vi "IKA_Eurostar60.vi"(5 "IKAenable":bool=TRUE, 6 "Timeout(s)":dbl=2.0, 7 "Command":T1, 8 "Error in":errorcluster, 9 "Set_parametro":dbl format="%.3f", 11 "VISA Paar mPDS2000":refnum<visa-resource-name>="ASRL6::INSTR") -> (0 "error out":errorcluster, 1 "Read_parametro":dbl format="%.3f", 2 "read string":string)   [LabVIEW 2017]
uses:
  IKA_Eurostar60.ctl
  <vilib>/Instr/_visa.llb/VISA Configure Serial Port (Instr).vi
panel:
  in  "EOS":string="\n"
  # "Input Data"
  # "Output Data"
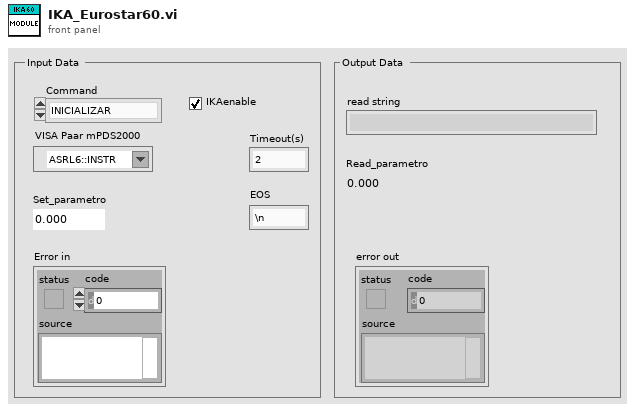
[diagram p1: front panel]
types:
  T1 = typedef "IKA_Eurostar60.ctl" = enum16{"INICIALIZAR", "READ NOMBRE APARATO", "READ VALOR PT100", "READ VELOCIDAD ACTUAL", "READ PAR DE GIRO ACTUAL", "READ VELOCIDAD NOMINAL", "READ LIMITE PAR DE GIRO", "READ LIMITE VELOCIDAD", "READ VELOCIDAD SEGURIDAD", "SET VELOCIDAD NOMINAL", "SET LIMITE PAR DE GIRO", "SET LIMITE VELOCIDAD", "SET VELOCIDAD SEGURIDAD", "ARRANCAR MOTOR", "DETENER MOTOR", "RESET", "SET SENTIDO DE GIRO", "READ SENTIDO DE GIRO", "FINALIZAR"}
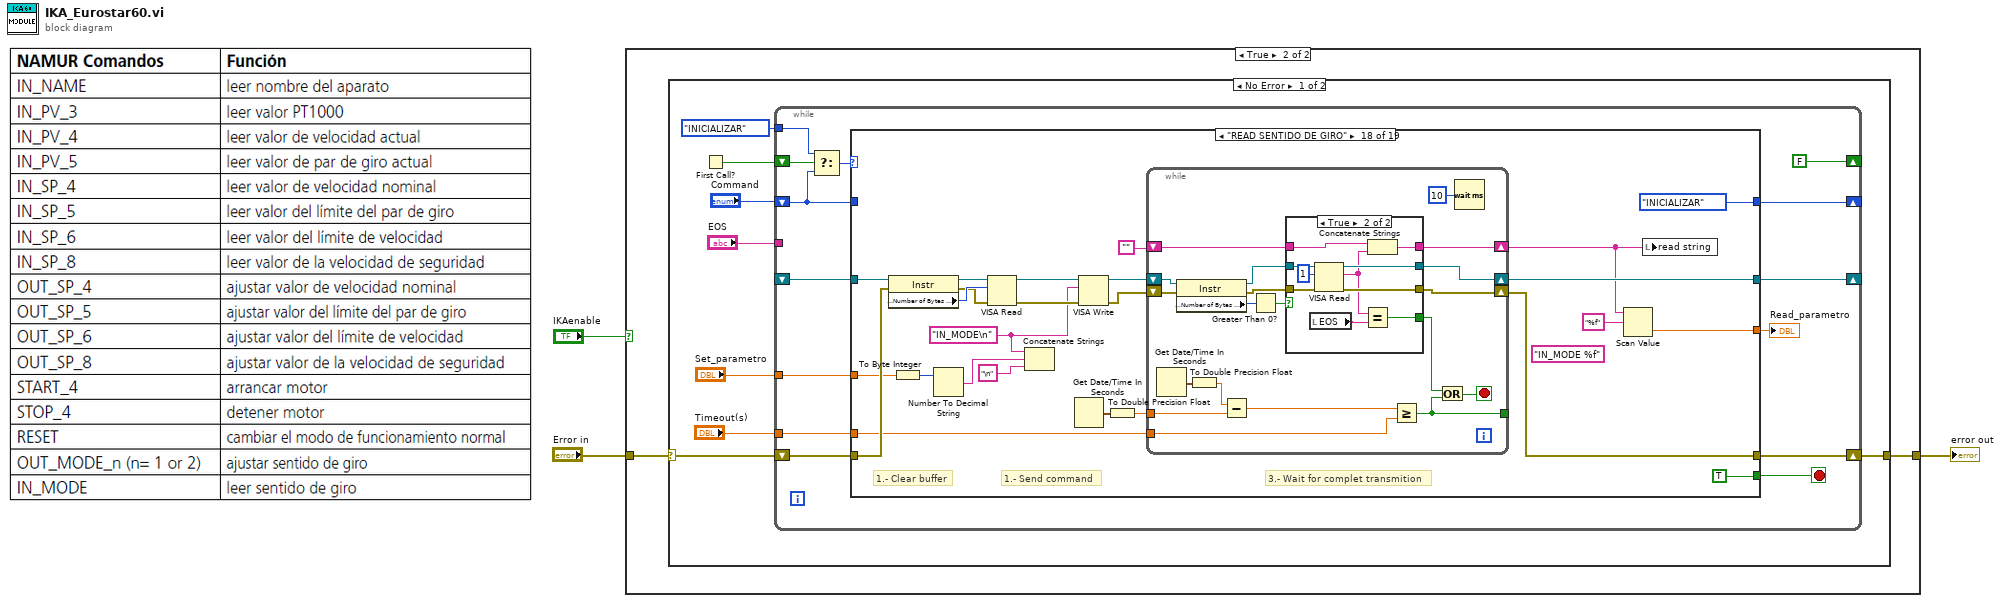
[diagram p0: block diagram]
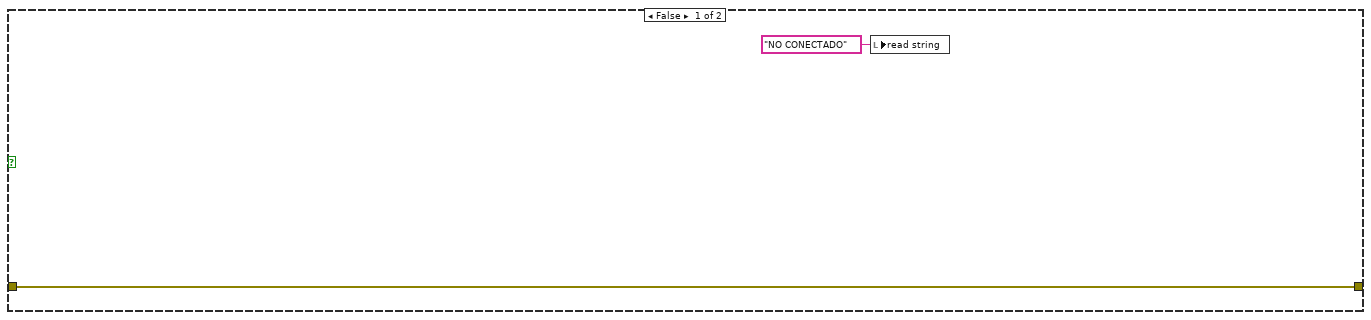
[diagram p2: hidden frame]
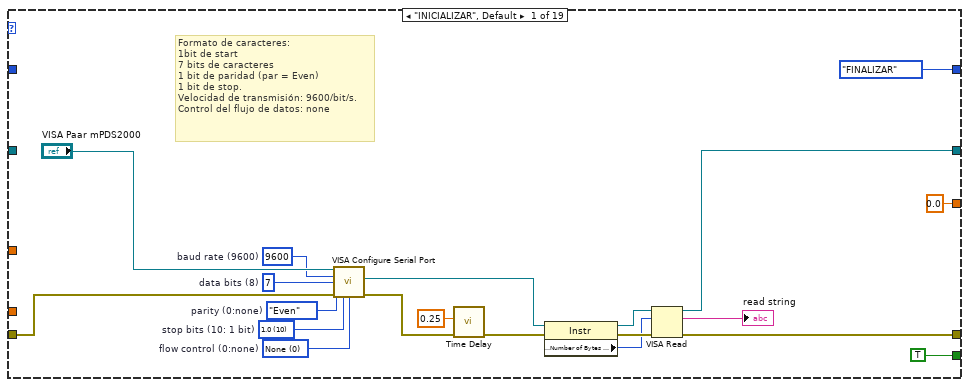
[diagram p3: hidden frame]
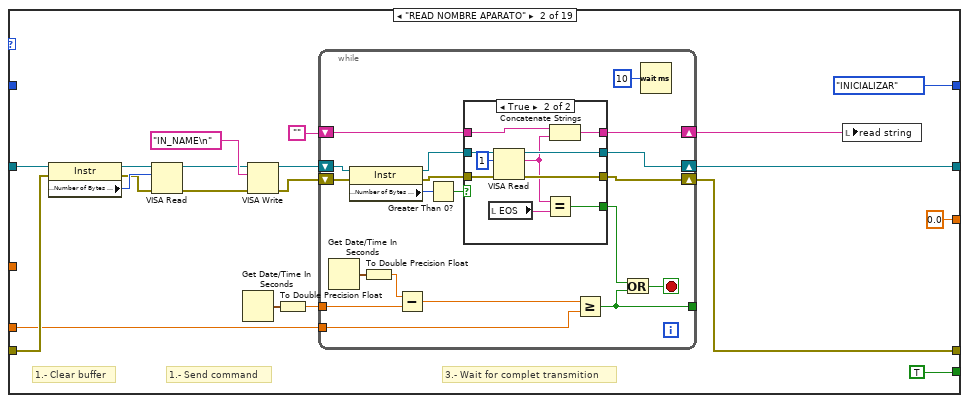
[diagram p4: hidden frame]
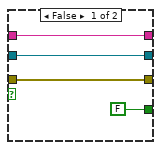
[diagram p5: hidden frame]
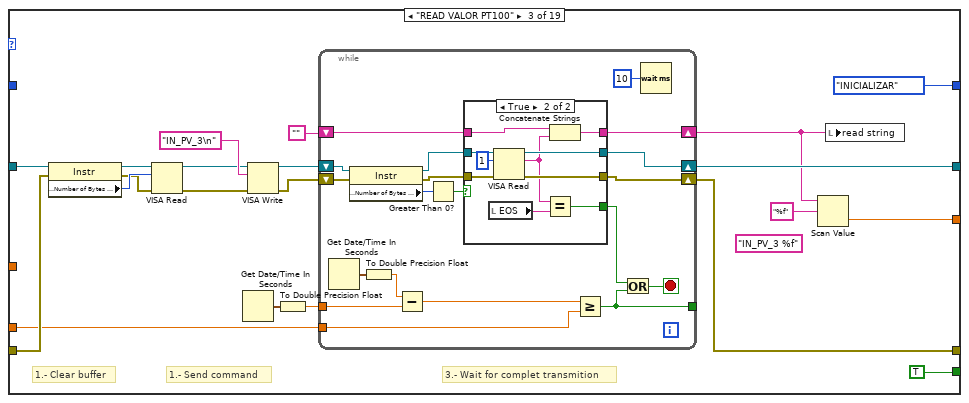
[diagram p6: hidden frame]
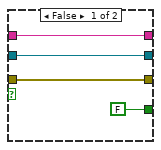
[diagram p7: hidden frame]
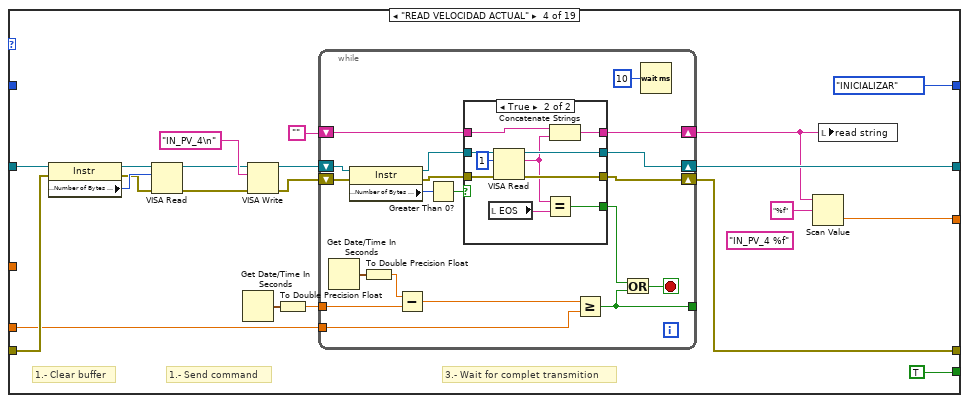
[diagram p8: hidden frame]
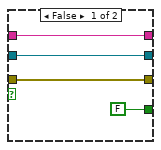
[diagram p9: hidden frame]
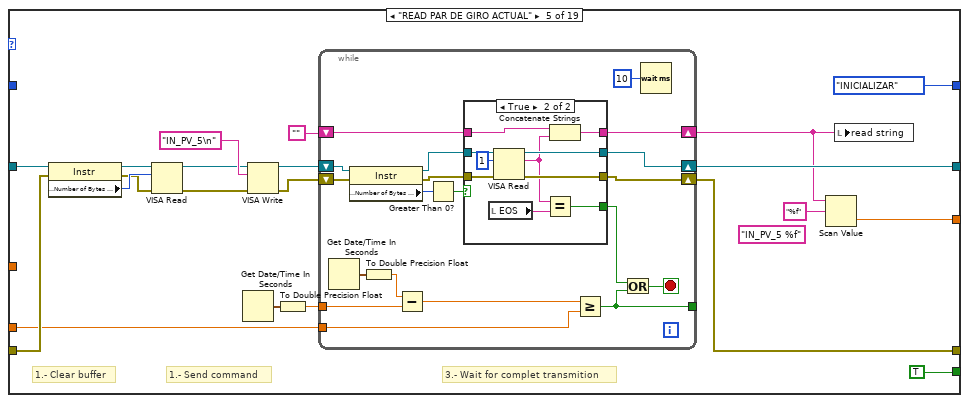
[diagram p10: hidden frame]
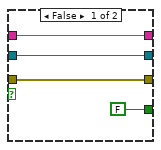
[diagram p11: hidden frame]
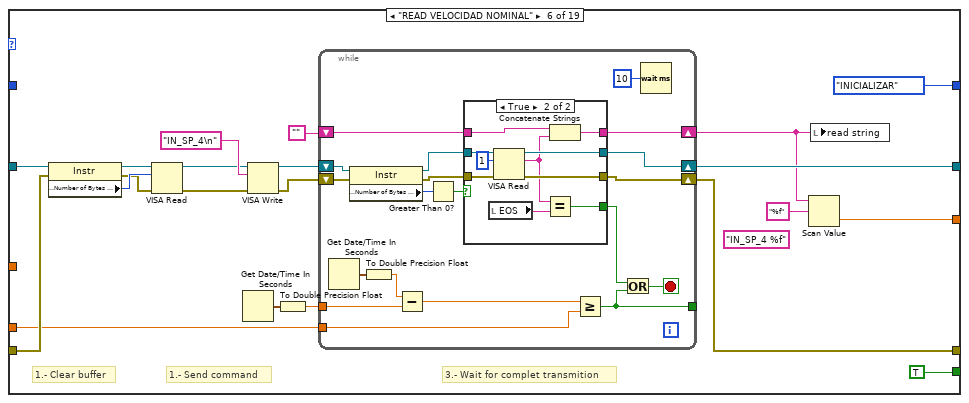
[diagram p12: hidden frame]
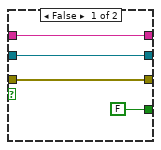
[diagram p13: hidden frame]
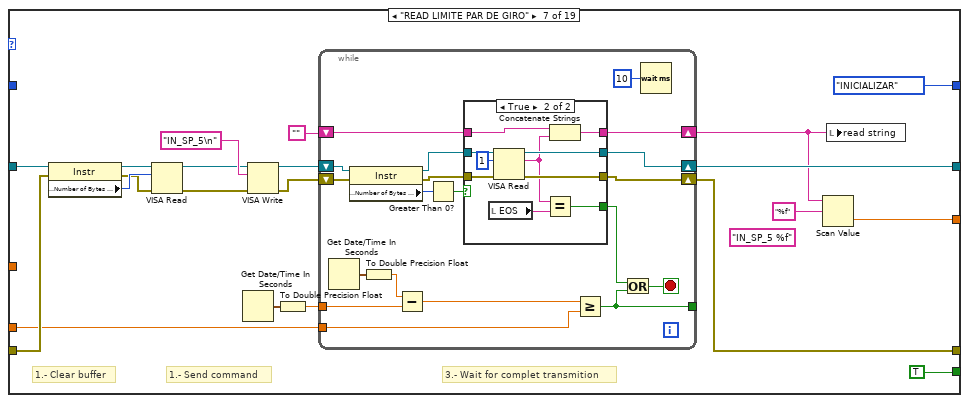
[diagram p14: hidden frame]
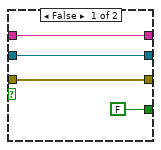
[diagram p15: hidden frame]
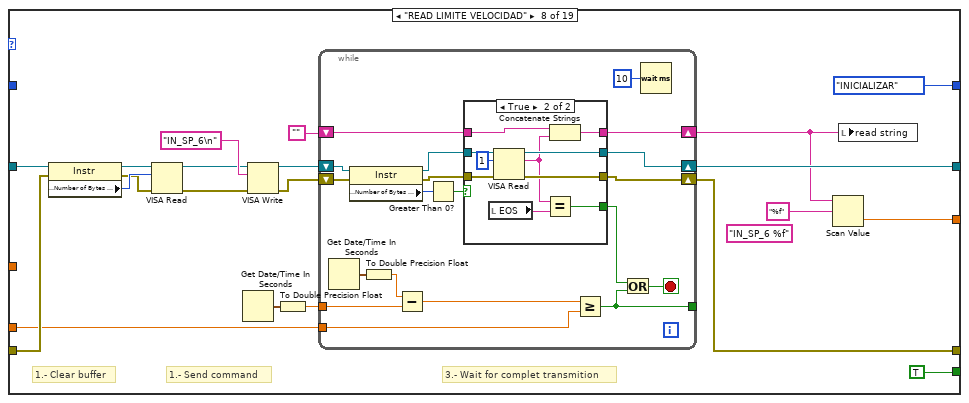
[diagram p16: hidden frame]
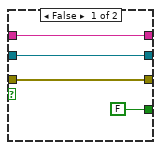
[diagram p17: hidden frame]
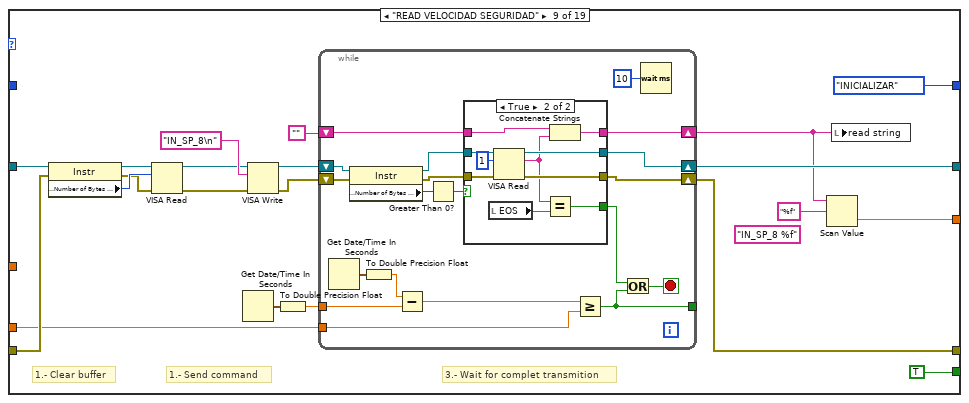
[diagram p18: hidden frame]
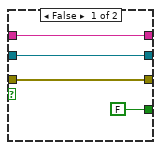
[diagram p19: hidden frame]
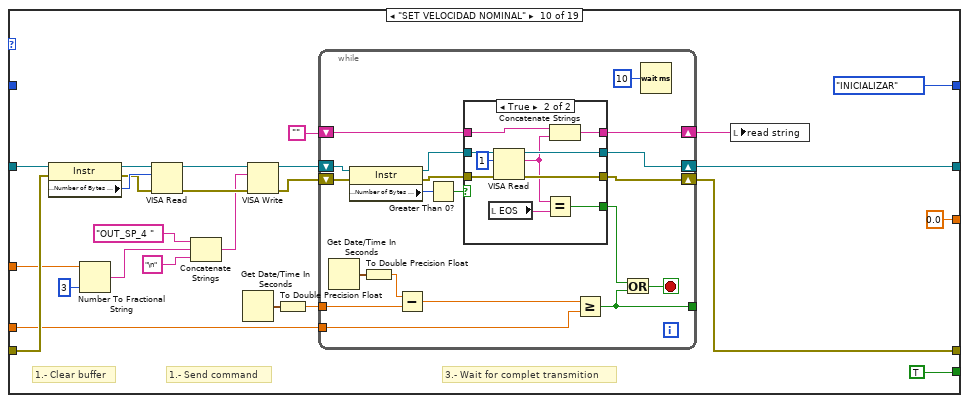
[diagram p20: hidden frame]
diagram:
  n1 = case shown="True" "IKAenable" {
    tunnel: "Error in" -> [w5 w7]
    tunnel: [w5 w6] -> w2
    frame False {
      n2 = local write "read string"("NO CONECTADO" ("read string")) -> ()
    }
    frame True {
      n3 = case shown="No Error" w7 {
        selector: w7 -> [w13 w1006]
        tunnel: [w12 w1006] -> w6
        frame No Error {
          n4 = First Call?() -> (First Call?: T/F=w15:bool)
          n5 = while {
            shift-right: [w21] -> _
            shift-left: "Command" -> [w22]
            shift-right: [w24] -> w12
            shift-left: w13 -> [w25]
            shift-right: [FALSE ("First Call?: T/F")] -> _
            shift-left: w15 -> [w29]
            tunnel: IKA_Eurostar60."INICIALIZAR" ("t") -> [w28]
            shift-right: [w19] -> _
            shift-left: _ -> [w20]
            tunnel: "Timeout(s)" -> [w18]
            tunnel: "Set_parametro" -> [w17]
            tunnel: "EOS" -> [_]
            stop <- w26 stop-if-true
            n6 = Select(t=w28, s=w29, f=w22) -> (s? t:f=w27:T1)
            n7 = case shown="\"READ SENTIDO DE GIRO\"" w27 {
              tunnel: [TRUE TRUE TRUE TRUE TRUE TRUE TRUE TRUE TRUE TRUE TRUE TRUE TRUE TRUE TRUE TRUE TRUE TRUE TRUE] -> w26
              tunnel: w25 -> [w46 w61 w115 w169 w223 w277 w331 w385 w439 w498 w556 w614 w672 w729 w786 w843 w901 w959 w1004]
              tunnel: [w48 w53 w107 w161 w215 w269 w323 w377 w431 w490 w548 w606 w664 w721 w778 w835 w893 w951 w1003] -> w24
              tunnel: w22 -> [_ _ _ _ _ _ _ _ _ _ _ _ _ _ _ _ _ _ _]
              tunnel: [IKA_Eurostar60."FINALIZAR" ("t") IKA_Eurostar60."INICIALIZAR" ("t") IKA_Eurostar60."INICIALIZAR" ("t") IKA_Eurostar60."INICIALIZAR" ("t") IKA_Eurostar60."INICIALIZAR" ("t") IKA_Eurostar60."INICIALIZAR" ("t") IKA_Eurostar60."INICIALIZAR" ("t") IKA_Eurostar60."INICIALIZAR" ("t") IKA_Eurostar60."INICIALIZAR" ("t") IKA_Eurostar60."INICIALIZAR" ("t") IKA_Eurostar60."INICIALIZAR" ("t") IKA_Eurostar60."INICIALIZAR" ("t") IKA_Eurostar60."INICIALIZAR" ("t") IKA_Eurostar60."INICIALIZAR" ("t") IKA_Eurostar60."INICIALIZAR" ("t") IKA_Eurostar60."INICIALIZAR" ("t") IKA_Eurostar60."INICIALIZAR" ("t") IKA_Eurostar60."INICIALIZAR" ("t") IKA_Eurostar60."FINALIZAR" ("t")] -> w21
              tunnel: w20 -> [_ w62 w116 w170 w224 w278 w332 w386 w440 w499 w557 w615 w673 w730 w787 w844 w902 w960 w1002]
              tunnel: [w47 w54 w108 w162 w216 w270 w324 w378 w432 w491 w549 w607 w665 w722 w779 w836 w894 w952 w1002] -> w19
              tunnel: w18 -> [_ w55 w109 w163 w217 w271 w325 w379 w433 w492 w550 w608 w666 w723 w780 w837 w895 w953 _]
              tunnel: w17 -> [_ _ _ _ _ _ _ _ _ w486 w544 w602 w660 w717 w774 w831 w888 w947 _]
              tunnel: [0.0 0.0 w103 w158 w211 w266 w321 w375 w427 0.0 0.0 0.0 0.0 0.0 0.0 0.0 0.0 w942 0.0] -> w16
              frame "INICIALIZAR", Default {
                w33 = u16 0 items=["None", "XON/XOFF", "RTS/CTS", "XON/XOFF & RTS/CTS", "DTR/DSR", "XON/XOFF & DTR/DSR"]  # flow control (0:none)
                w34 = u16 10 items=["1.0"=10, "1.5"=15, "2.0"=20]  # stop bits (10: 1 bit)
                w35 = enum16{"None", "Odd", "Even", "Mark", "Space"}."Even"  # parity (0:none)
                w36 = u16 7  # data bits (8)
                w37 = u32 9600  # baud rate (9600)
                # "Formato de caracteres: \n1bit de start\n7 bits de caracteres\n1 bit de paridad (par = Even)\n1 bit de stop.\nVelocidad de transmisión: 9600/bit/s.\nControl del flujo de datos: none"
                n8 = call-poly "VISA Configure Serial Port"("VISA resource name"="VISA Paar mPDS2000", "baud rate (9600)"=w37, "data bits (8)"=w36, "parity (0:none)"=w35, "error in (no error)"=w46, "stop bits (10: 1 bit)"=w34, "flow control (0:none)"=w33) -> ("VISA resource name out"=w41:refnum<visa-resource-name>, "error out"=w39:errorcluster)  [unwired: 7 in]
                n9 = call "Time Delay"("error in (no error)"=w39, "Delay Time (s)"=0.25) -> ("error out"=w38:errorcluster)  [unwired: 9 in]
                n10 = property class="Instr"(reference=w41, error in=w38) -> (reference out=w44:refnum<visa-resource-name>, error out=w43:errorcluster, "Serial Settings:Number of Bytes at Serial Port"=w42:u32)
                n11 = VISA Read(VISA resource name=w44, byte count=w42, error in (no error)=w43) -> (VISA resource name out=w47:refnum<visa-resource-name>, read buffer=→"read string":string, error out=w48:errorcluster)  [unwired: 1 out]
              }
              frame "READ NOMBRE APARATO" {
                # "1.- Send command"
                # "3.- Wait for complet transmition"
                # "1.- Clear buffer"
                n12 = property class="Instr"(reference=w62, error in=w61) -> (reference out=w65:refnum<visa-resource-name>, error out=w66:errorcluster, "Serial Settings:Number of Bytes at Serial Port"=w67:u32)
                n13 = VISA Read(VISA resource name=w65, byte count=w67, error in (no error)=w66) -> (VISA resource name out=w64:refnum<visa-resource-name>, error out=w63:errorcluster)  [unwired: 2 out]
                n14 = Get Date/Time In Seconds() -> (seconds since 1Jan1904=w59:timestamp)
                n15 = VISA Write(VISA resource name=w64, write buffer="IN_NAME\n" ("Mide"), error in (no error)=w63) -> (VISA resource name out=w57:refnum<visa-resource-name>, error out=w56:errorcluster)  [unwired: 1 out]
                n16 = To Double Precision Float(number=w59) -> (double precision float=w58:dbl)
                n17 = while {
                  tunnel: w58 -> [w85]
                  shift-right: [w73] -> w54
                  shift-left: w57 -> [w84]
                  shift-right: [w72] -> w53
                  shift-left: w56 -> [w83]
                  tunnel: w55 -> [w81]
                  tunnel: [w80] -> _
                  shift-right: [w76] -> w51
                  shift-left: "" -> [w71]
                  stop <- w88 stop-if-true
                  n18 = Get Date/Time In Seconds() -> (seconds since 1Jan1904=w87:timestamp)
                  n19 = property class="Instr"(reference=w84, error in=w83) -> (reference out=w74:refnum<visa-resource-name>, error out=w75:errorcluster, "Serial Settings:Number of Bytes at Serial Port"=w78:u32)
                  n20 = To Double Precision Float(number=w87) -> (double precision float=w86:dbl)
                  n21 = Subtract(x=w86, y=w85) -> (x-y=w82:dbl)
                  n22 = Greater Than 0?(x=w78) -> (x > 0?=w77:bool)
                  n23 = case shown="True" w77 {
                    tunnel: w71 -> [w92 w97]
                    tunnel: [w92 w96] -> w76
                    tunnel: w75 -> [w90 w102]
                    tunnel: w74 -> [w89 w101]
                    tunnel: [w89 w100] -> w73
                    tunnel: [w90 w99] -> w72
                    tunnel: [FALSE w94] -> w70
                    frame False {
                    }
                    frame True {
                      n24 = local read "EOS"() -> (w93:string)
                      n25 = VISA Read(VISA resource name=w101, byte count=u32 1, error in (no error)=w102) -> (VISA resource name out=w100:refnum<visa-resource-name>, read buffer=w95:string, error out=w99:errorcluster)  [unwired: 1 out]
                      n26 = Equal?(x=w95, y=w93) -> (x = y?=w94:bool)
                      n27 = Concatenate Strings(w97, w95) -> (w96:string)
                    }
                  }
                  n28 = Greater Or Equal?(x=w82, y=w81) -> (x >= y?=w80:bool)
                  n29 = Or(x=w70, y=w80) -> (x .or. y?=w88:bool)
                  n30 = Wait (ms)(milliseconds to wait=u32 10) -> ()  [unwired: 1 out]
                }
                n31 = local write "read string"(w51) -> ()
              }
              frame "READ VALOR PT100" {
                (unwired) "IN_PV_3 %f" ("format string")
                # "1.- Send command"
                # "3.- Wait for complet transmition"
                # "1.- Clear buffer"
                n32 = property class="Instr"(reference=w116, error in=w115) -> (reference out=w119:refnum<visa-resource-name>, error out=w120:errorcluster, "Serial Settings:Number of Bytes at Serial Port"=w121:u32)
                n33 = VISA Read(VISA resource name=w119, byte count=w121, error in (no error)=w120) -> (VISA resource name out=w118:refnum<visa-resource-name>, error out=w117:errorcluster)  [unwired: 2 out]
                n34 = Get Date/Time In Seconds() -> (seconds since 1Jan1904=w113:timestamp)
                n35 = VISA Write(VISA resource name=w118, write buffer="IN_PV_3\n" ("Mide"), error in (no error)=w117) -> (VISA resource name out=w111:refnum<visa-resource-name>, error out=w110:errorcluster)  [unwired: 1 out]
                n36 = To Double Precision Float(number=w113) -> (double precision float=w112:dbl)
                n37 = while {
                  tunnel: w112 -> [w139]
                  shift-right: [w127] -> w108
                  shift-left: w111 -> [w138]
                  shift-right: [w126] -> w107
                  shift-left: w110 -> [w137]
                  tunnel: w109 -> [w135]
                  tunnel: [w134] -> _
                  shift-right: [w130] -> w104
                  shift-left: "" -> [w125]
                  stop <- w142 stop-if-true
                  n38 = Get Date/Time In Seconds() -> (seconds since 1Jan1904=w141:timestamp)
                  n39 = property class="Instr"(reference=w138, error in=w137) -> (reference out=w128:refnum<visa-resource-name>, error out=w129:errorcluster, "Serial Settings:Number of Bytes at Serial Port"=w132:u32)
                  n40 = To Double Precision Float(number=w141) -> (double precision float=w140:dbl)
                  n41 = Subtract(x=w140, y=w139) -> (x-y=w136:dbl)
                  n42 = Greater Than 0?(x=w132) -> (x > 0?=w131:bool)
                  n43 = case shown="True" w131 {
                    tunnel: w125 -> [w146 w151]
                    tunnel: [w146 w150] -> w130
                    tunnel: w129 -> [w144 w156]
                    tunnel: w128 -> [w143 w155]
                    tunnel: [w143 w154] -> w127
                    tunnel: [w144 w153] -> w126
                    tunnel: [FALSE w148] -> w124
                    frame False {
                    }
                    frame True {
                      n44 = local read "EOS"() -> (w147:string)
                      n45 = VISA Read(VISA resource name=w155, byte count=u32 1, error in (no error)=w156) -> (VISA resource name out=w154:refnum<visa-resource-name>, read buffer=w149:string, error out=w153:errorcluster)  [unwired: 1 out]
                      n46 = Equal?(x=w149, y=w147) -> (x = y?=w148:bool)
                      n47 = Concatenate Strings(w151, w149) -> (w150:string)
                    }
                  }
                  n48 = Greater Or Equal?(x=w136, y=w135) -> (x >= y?=w134:bool)
                  n49 = Or(x=w124, y=w134) -> (x .or. y?=w142:bool)
                  n50 = Wait (ms)(milliseconds to wait=u32 10) -> ()  [unwired: 1 out]
                }
                n51 = Scan Value(string=w104, format string="%f") -> (value=w103:dbl)  [unwired: 1 in, 1 out]
                n52 = local write "read string"(w104) -> ()
              }
              frame "READ VELOCIDAD ACTUAL" {
                (unwired) "IN_PV_4 %f" ("format string")
                # "1.- Send command"
                # "3.- Wait for complet transmition"
                # "1.- Clear buffer"
                n53 = property class="Instr"(reference=w170, error in=w169) -> (reference out=w173:refnum<visa-resource-name>, error out=w174:errorcluster, "Serial Settings:Number of Bytes at Serial Port"=w175:u32)
                n54 = VISA Read(VISA resource name=w173, byte count=w175, error in (no error)=w174) -> (VISA resource name out=w172:refnum<visa-resource-name>, error out=w171:errorcluster)  [unwired: 2 out]
                n55 = Get Date/Time In Seconds() -> (seconds since 1Jan1904=w167:timestamp)
                n56 = VISA Write(VISA resource name=w172, write buffer="IN_PV_4\n" ("Mide"), error in (no error)=w171) -> (VISA resource name out=w165:refnum<visa-resource-name>, error out=w164:errorcluster)  [unwired: 1 out]
                n57 = To Double Precision Float(number=w167) -> (double precision float=w166:dbl)
                n58 = while {
                  tunnel: w166 -> [w193]
                  shift-right: [w181] -> w162
                  shift-left: w165 -> [w192]
                  shift-right: [w180] -> w161
                  shift-left: w164 -> [w191]
                  tunnel: w163 -> [w189]
                  tunnel: [w188] -> _
                  shift-right: [w184] -> w157
                  shift-left: "" -> [w179]
                  stop <- w196 stop-if-true
                  n59 = Get Date/Time In Seconds() -> (seconds since 1Jan1904=w195:timestamp)
                  n60 = property class="Instr"(reference=w192, error in=w191) -> (reference out=w182:refnum<visa-resource-name>, error out=w183:errorcluster, "Serial Settings:Number of Bytes at Serial Port"=w186:u32)
                  n61 = To Double Precision Float(number=w195) -> (double precision float=w194:dbl)
                  n62 = Subtract(x=w194, y=w193) -> (x-y=w190:dbl)
                  n63 = Greater Than 0?(x=w186) -> (x > 0?=w185:bool)
                  n64 = case shown="True" w185 {
                    tunnel: w179 -> [w200 w205]
                    tunnel: [w200 w204] -> w184
                    tunnel: w183 -> [w198 w210]
                    tunnel: w182 -> [w197 w209]
                    tunnel: [w197 w208] -> w181
                    tunnel: [w198 w207] -> w180
                    tunnel: [FALSE w202] -> w178
                    frame False {
                    }
                    frame True {
                      n65 = local read "EOS"() -> (w201:string)
                      n66 = VISA Read(VISA resource name=w209, byte count=u32 1, error in (no error)=w210) -> (VISA resource name out=w208:refnum<visa-resource-name>, read buffer=w203:string, error out=w207:errorcluster)  [unwired: 1 out]
                      n67 = Equal?(x=w203, y=w201) -> (x = y?=w202:bool)
                      n68 = Concatenate Strings(w205, w203) -> (w204:string)
                    }
                  }
                  n69 = Greater Or Equal?(x=w190, y=w189) -> (x >= y?=w188:bool)
                  n70 = Or(x=w178, y=w188) -> (x .or. y?=w196:bool)
                  n71 = Wait (ms)(milliseconds to wait=u32 10) -> ()  [unwired: 1 out]
                }
                n72 = Scan Value(string=w157, format string="%f") -> (value=w158:dbl)  [unwired: 1 in, 1 out]
                n73 = local write "read string"(w157) -> ()
              }
              frame "READ PAR DE GIRO ACTUAL" {
                (unwired) "IN_PV_5 %f" ("format string")
                # "1.- Send command"
                # "3.- Wait for complet transmition"
                # "1.- Clear buffer"
                n74 = property class="Instr"(reference=w224, error in=w223) -> (reference out=w227:refnum<visa-resource-name>, error out=w228:errorcluster, "Serial Settings:Number of Bytes at Serial Port"=w229:u32)
                n75 = VISA Read(VISA resource name=w227, byte count=w229, error in (no error)=w228) -> (VISA resource name out=w226:refnum<visa-resource-name>, error out=w225:errorcluster)  [unwired: 2 out]
                n76 = Get Date/Time In Seconds() -> (seconds since 1Jan1904=w221:timestamp)
                n77 = VISA Write(VISA resource name=w226, write buffer="IN_PV_5\n" ("Mide"), error in (no error)=w225) -> (VISA resource name out=w219:refnum<visa-resource-name>, error out=w218:errorcluster)  [unwired: 1 out]
                n78 = To Double Precision Float(number=w221) -> (double precision float=w220:dbl)
                n79 = while {
                  tunnel: w220 -> [w247]
                  shift-right: [w235] -> w216
                  shift-left: w219 -> [w246]
                  shift-right: [w234] -> w215
                  shift-left: w218 -> [w245]
                  tunnel: w217 -> [w243]
                  tunnel: [w242] -> _
                  shift-right: [w238] -> w212
                  shift-left: "" -> [w233]
                  stop <- w250 stop-if-true
                  n80 = Get Date/Time In Seconds() -> (seconds since 1Jan1904=w249:timestamp)
                  n81 = property class="Instr"(reference=w246, error in=w245) -> (reference out=w236:refnum<visa-resource-name>, error out=w237:errorcluster, "Serial Settings:Number of Bytes at Serial Port"=w240:u32)
                  n82 = To Double Precision Float(number=w249) -> (double precision float=w248:dbl)
                  n83 = Subtract(x=w248, y=w247) -> (x-y=w244:dbl)
                  n84 = Greater Than 0?(x=w240) -> (x > 0?=w239:bool)
                  n85 = case shown="True" w239 {
                    tunnel: w233 -> [w254 w259]
                    tunnel: [w254 w258] -> w238
                    tunnel: w237 -> [w252 w264]
                    tunnel: w236 -> [w251 w263]
                    tunnel: [w251 w262] -> w235
                    tunnel: [w252 w261] -> w234
                    tunnel: [FALSE w256] -> w232
                    frame False {
                    }
                    frame True {
                      n86 = local read "EOS"() -> (w255:string)
                      n87 = VISA Read(VISA resource name=w263, byte count=u32 1, error in (no error)=w264) -> (VISA resource name out=w262:refnum<visa-resource-name>, read buffer=w257:string, error out=w261:errorcluster)  [unwired: 1 out]
                      n88 = Equal?(x=w257, y=w255) -> (x = y?=w256:bool)
                      n89 = Concatenate Strings(w259, w257) -> (w258:string)
                    }
                  }
                  n90 = Greater Or Equal?(x=w244, y=w243) -> (x >= y?=w242:bool)
                  n91 = Or(x=w232, y=w242) -> (x .or. y?=w250:bool)
                  n92 = Wait (ms)(milliseconds to wait=u32 10) -> ()  [unwired: 1 out]
                }
                n93 = Scan Value(string=w212, format string="%f") -> (value=w211:dbl)  [unwired: 1 in, 1 out]
                n94 = local write "read string"(w212) -> ()
              }
              frame "READ VELOCIDAD NOMINAL" {
                (unwired) "IN_SP_4 %f" ("format string")
                # "1.- Send command"
                # "3.- Wait for complet transmition"
                # "1.- Clear buffer"
                n95 = property class="Instr"(reference=w278, error in=w277) -> (reference out=w281:refnum<visa-resource-name>, error out=w282:errorcluster, "Serial Settings:Number of Bytes at Serial Port"=w283:u32)
                n96 = VISA Read(VISA resource name=w281, byte count=w283, error in (no error)=w282) -> (VISA resource name out=w280:refnum<visa-resource-name>, error out=w279:errorcluster)  [unwired: 2 out]
                n97 = Get Date/Time In Seconds() -> (seconds since 1Jan1904=w275:timestamp)
                n98 = VISA Write(VISA resource name=w280, write buffer="IN_SP_4\n" ("Mide"), error in (no error)=w279) -> (VISA resource name out=w273:refnum<visa-resource-name>, error out=w272:errorcluster)  [unwired: 1 out]
                n99 = To Double Precision Float(number=w275) -> (double precision float=w274:dbl)
                n100 = while {
                  tunnel: w274 -> [w301]
                  shift-right: [w289] -> w270
                  shift-left: w273 -> [w300]
                  shift-right: [w288] -> w269
                  shift-left: w272 -> [w299]
                  tunnel: w271 -> [w297]
                  tunnel: [w296] -> _
                  shift-right: [w292] -> w265
                  shift-left: "" -> [w287]
                  stop <- w304 stop-if-true
                  n101 = Get Date/Time In Seconds() -> (seconds since 1Jan1904=w303:timestamp)
                  n102 = property class="Instr"(reference=w300, error in=w299) -> (reference out=w290:refnum<visa-resource-name>, error out=w291:errorcluster, "Serial Settings:Number of Bytes at Serial Port"=w294:u32)
                  n103 = To Double Precision Float(number=w303) -> (double precision float=w302:dbl)
                  n104 = Subtract(x=w302, y=w301) -> (x-y=w298:dbl)
                  n105 = Greater Than 0?(x=w294) -> (x > 0?=w293:bool)
                  n106 = case shown="True" w293 {
                    tunnel: w287 -> [w308 w313]
                    tunnel: [w308 w312] -> w292
                    tunnel: w291 -> [w306 w318]
                    tunnel: w290 -> [w305 w317]
                    tunnel: [w305 w316] -> w289
                    tunnel: [w306 w315] -> w288
                    tunnel: [FALSE w310] -> w286
                    frame False {
                    }
                    frame True {
                      n107 = local read "EOS"() -> (w309:string)
                      n108 = VISA Read(VISA resource name=w317, byte count=u32 1, error in (no error)=w318) -> (VISA resource name out=w316:refnum<visa-resource-name>, read buffer=w311:string, error out=w315:errorcluster)  [unwired: 1 out]
                      n109 = Equal?(x=w311, y=w309) -> (x = y?=w310:bool)
                      n110 = Concatenate Strings(w313, w311) -> (w312:string)
                    }
                  }
                  n111 = Greater Or Equal?(x=w298, y=w297) -> (x >= y?=w296:bool)
                  n112 = Or(x=w286, y=w296) -> (x .or. y?=w304:bool)
                  n113 = Wait (ms)(milliseconds to wait=u32 10) -> ()  [unwired: 1 out]
                }
                n114 = Scan Value(string=w265, format string="%f") -> (value=w266:dbl)  [unwired: 1 in, 1 out]
                n115 = local write "read string"(w265) -> ()
              }
              frame "READ LIMITE PAR DE GIRO" {
                (unwired) "IN_SP_5 %f" ("format string")
                # "1.- Send command"
                # "3.- Wait for complet transmition"
                # "1.- Clear buffer"
                n116 = property class="Instr"(reference=w332, error in=w331) -> (reference out=w335:refnum<visa-resource-name>, error out=w336:errorcluster, "Serial Settings:Number of Bytes at Serial Port"=w337:u32)
                n117 = VISA Read(VISA resource name=w335, byte count=w337, error in (no error)=w336) -> (VISA resource name out=w334:refnum<visa-resource-name>, error out=w333:errorcluster)  [unwired: 2 out]
                n118 = Get Date/Time In Seconds() -> (seconds since 1Jan1904=w329:timestamp)
                n119 = VISA Write(VISA resource name=w334, write buffer="IN_SP_5\n" ("Mide"), error in (no error)=w333) -> (VISA resource name out=w327:refnum<visa-resource-name>, error out=w326:errorcluster)  [unwired: 1 out]
                n120 = To Double Precision Float(number=w329) -> (double precision float=w328:dbl)
                n121 = while {
                  tunnel: w328 -> [w355]
                  shift-right: [w343] -> w324
                  shift-left: w327 -> [w354]
                  shift-right: [w342] -> w323
                  shift-left: w326 -> [w353]
                  tunnel: w325 -> [w351]
                  tunnel: [w350] -> _
                  shift-right: [w346] -> w320
                  shift-left: "" -> [w341]
                  stop <- w358 stop-if-true
                  n122 = Get Date/Time In Seconds() -> (seconds since 1Jan1904=w357:timestamp)
                  n123 = property class="Instr"(reference=w354, error in=w353) -> (reference out=w344:refnum<visa-resource-name>, error out=w345:errorcluster, "Serial Settings:Number of Bytes at Serial Port"=w348:u32)
                  n124 = To Double Precision Float(number=w357) -> (double precision float=w356:dbl)
                  n125 = Subtract(x=w356, y=w355) -> (x-y=w352:dbl)
                  n126 = Greater Than 0?(x=w348) -> (x > 0?=w347:bool)
                  n127 = case shown="True" w347 {
                    tunnel: w341 -> [w362 w367]
                    tunnel: [w362 w366] -> w346
                    tunnel: w345 -> [w360 w372]
                    tunnel: w344 -> [w359 w371]
                    tunnel: [w359 w370] -> w343
                    tunnel: [w360 w369] -> w342
                    tunnel: [FALSE w364] -> w340
                    frame False {
                    }
                    frame True {
                      n128 = local read "EOS"() -> (w363:string)
                      n129 = VISA Read(VISA resource name=w371, byte count=u32 1, error in (no error)=w372) -> (VISA resource name out=w370:refnum<visa-resource-name>, read buffer=w365:string, error out=w369:errorcluster)  [unwired: 1 out]
                      n130 = Equal?(x=w365, y=w363) -> (x = y?=w364:bool)
                      n131 = Concatenate Strings(w367, w365) -> (w366:string)
                    }
                  }
                  n132 = Greater Or Equal?(x=w352, y=w351) -> (x >= y?=w350:bool)
                  n133 = Or(x=w340, y=w350) -> (x .or. y?=w358:bool)
                  n134 = Wait (ms)(milliseconds to wait=u32 10) -> ()  [unwired: 1 out]
                }
                n135 = Scan Value(string=w320, format string="%f") -> (value=w321:dbl)  [unwired: 1 in, 1 out]
                n136 = local write "read string"(w320) -> ()
              }
              frame "READ LIMITE VELOCIDAD" {
                (unwired) "IN_SP_6 %f" ("format string")
                # "1.- Send command"
                # "3.- Wait for complet transmition"
                # "1.- Clear buffer"
                n137 = property class="Instr"(reference=w386, error in=w385) -> (reference out=w389:refnum<visa-resource-name>, error out=w390:errorcluster, "Serial Settings:Number of Bytes at Serial Port"=w391:u32)
                n138 = VISA Read(VISA resource name=w389, byte count=w391, error in (no error)=w390) -> (VISA resource name out=w388:refnum<visa-resource-name>, error out=w387:errorcluster)  [unwired: 2 out]
                n139 = Get Date/Time In Seconds() -> (seconds since 1Jan1904=w383:timestamp)
                n140 = VISA Write(VISA resource name=w388, write buffer="IN_SP_6\n" ("Mide"), error in (no error)=w387) -> (VISA resource name out=w381:refnum<visa-resource-name>, error out=w380:errorcluster)  [unwired: 1 out]
                n141 = To Double Precision Float(number=w383) -> (double precision float=w382:dbl)
                n142 = while {
                  tunnel: w382 -> [w409]
                  shift-right: [w397] -> w378
                  shift-left: w381 -> [w408]
                  shift-right: [w396] -> w377
                  shift-left: w380 -> [w407]
                  tunnel: w379 -> [w405]
                  tunnel: [w404] -> _
                  shift-right: [w400] -> w373
                  shift-left: "" -> [w395]
                  stop <- w412 stop-if-true
                  n143 = Get Date/Time In Seconds() -> (seconds since 1Jan1904=w411:timestamp)
                  n144 = property class="Instr"(reference=w408, error in=w407) -> (reference out=w398:refnum<visa-resource-name>, error out=w399:errorcluster, "Serial Settings:Number of Bytes at Serial Port"=w402:u32)
                  n145 = To Double Precision Float(number=w411) -> (double precision float=w410:dbl)
                  n146 = Subtract(x=w410, y=w409) -> (x-y=w406:dbl)
                  n147 = Greater Than 0?(x=w402) -> (x > 0?=w401:bool)
                  n148 = case shown="True" w401 {
                    tunnel: w395 -> [w416 w421]
                    tunnel: [w416 w420] -> w400
                    tunnel: w399 -> [w414 w426]
                    tunnel: w398 -> [w413 w425]
                    tunnel: [w413 w424] -> w397
                    tunnel: [w414 w423] -> w396
                    tunnel: [FALSE w418] -> w394
                    frame False {
                    }
                    frame True {
                      n149 = local read "EOS"() -> (w417:string)
                      n150 = VISA Read(VISA resource name=w425, byte count=u32 1, error in (no error)=w426) -> (VISA resource name out=w424:refnum<visa-resource-name>, read buffer=w419:string, error out=w423:errorcluster)  [unwired: 1 out]
                      n151 = Equal?(x=w419, y=w417) -> (x = y?=w418:bool)
                      n152 = Concatenate Strings(w421, w419) -> (w420:string)
                    }
                  }
                  n153 = Greater Or Equal?(x=w406, y=w405) -> (x >= y?=w404:bool)
                  n154 = Or(x=w394, y=w404) -> (x .or. y?=w412:bool)
                  n155 = Wait (ms)(milliseconds to wait=u32 10) -> ()  [unwired: 1 out]
                }
                n156 = Scan Value(string=w373, format string="%f") -> (value=w375:dbl)  [unwired: 1 in, 1 out]
                n157 = local write "read string"(w373) -> ()
              }
              frame "READ VELOCIDAD SEGURIDAD" {
                (unwired) "IN_SP_8 %f" ("format string")
                # "1.- Send command"
                # "3.- Wait for complet transmition"
                # "1.- Clear buffer"
                n158 = property class="Instr"(reference=w440, error in=w439) -> (reference out=w443:refnum<visa-resource-name>, error out=w444:errorcluster, "Serial Settings:Number of Bytes at Serial Port"=w445:u32)
                n159 = VISA Read(VISA resource name=w443, byte count=w445, error in (no error)=w444) -> (VISA resource name out=w442:refnum<visa-resource-name>, error out=w441:errorcluster)  [unwired: 2 out]
                n160 = Get Date/Time In Seconds() -> (seconds since 1Jan1904=w437:timestamp)
                n161 = VISA Write(VISA resource name=w442, write buffer="IN_SP_8\n" ("Mide"), error in (no error)=w441) -> (VISA resource name out=w435:refnum<visa-resource-name>, error out=w434:errorcluster)  [unwired: 1 out]
                n162 = To Double Precision Float(number=w437) -> (double precision float=w436:dbl)
                n163 = while {
                  tunnel: w436 -> [w463]
                  shift-right: [w451] -> w432
                  shift-left: w435 -> [w462]
                  shift-right: [w450] -> w431
                  shift-left: w434 -> [w461]
                  tunnel: w433 -> [w459]
                  tunnel: [w458] -> _
                  shift-right: [w454] -> w428
                  shift-left: "" -> [w449]
                  stop <- w466 stop-if-true
                  n164 = Get Date/Time In Seconds() -> (seconds since 1Jan1904=w465:timestamp)
                  n165 = property class="Instr"(reference=w462, error in=w461) -> (reference out=w452:refnum<visa-resource-name>, error out=w453:errorcluster, "Serial Settings:Number of Bytes at Serial Port"=w456:u32)
                  n166 = To Double Precision Float(number=w465) -> (double precision float=w464:dbl)
                  n167 = Subtract(x=w464, y=w463) -> (x-y=w460:dbl)
                  n168 = Greater Than 0?(x=w456) -> (x > 0?=w455:bool)
                  n169 = case shown="True" w455 {
                    tunnel: w449 -> [w470 w475]
                    tunnel: [w470 w474] -> w454
                    tunnel: w453 -> [w468 w480]
                    tunnel: w452 -> [w467 w479]
                    tunnel: [w467 w478] -> w451
                    tunnel: [w468 w477] -> w450
                    tunnel: [FALSE w472] -> w448
                    frame False {
                    }
                    frame True {
                      n170 = local read "EOS"() -> (w471:string)
                      n171 = VISA Read(VISA resource name=w479, byte count=u32 1, error in (no error)=w480) -> (VISA resource name out=w478:refnum<visa-resource-name>, read buffer=w473:string, error out=w477:errorcluster)  [unwired: 1 out]
                      n172 = Equal?(x=w473, y=w471) -> (x = y?=w472:bool)
                      n173 = Concatenate Strings(w475, w473) -> (w474:string)
                    }
                  }
                  n174 = Greater Or Equal?(x=w460, y=w459) -> (x >= y?=w458:bool)
                  n175 = Or(x=w448, y=w458) -> (x .or. y?=w466:bool)
                  n176 = Wait (ms)(milliseconds to wait=u32 10) -> ()  [unwired: 1 out]
                }
                n177 = Scan Value(string=w428, format string="%f") -> (value=w427:dbl)  [unwired: 1 in, 1 out]
                n178 = local write "read string"(w428) -> ()
              }
              frame "SET VELOCIDAD NOMINAL" {
                # "1.- Send command"
                # "3.- Wait for complet transmition"
                # "1.- Clear buffer"
                n179 = property class="Instr"(reference=w499, error in=w498) -> (reference out=w502:refnum<visa-resource-name>, error out=w503:errorcluster, "Serial Settings:Number of Bytes at Serial Port"=w504:u32)
                n180 = Number To Fractional String(number=w486, precision (6)=i16 3) -> (F-format string=w483:string)  [unwired: 2 in]
                n181 = VISA Read(VISA resource name=w502, byte count=w504, error in (no error)=w503) -> (VISA resource name out=w501:refnum<visa-resource-name>, error out=w500:errorcluster)  [unwired: 2 out]
                n182 = Concatenate Strings("OUT_SP_4 " ("Mide"), w483, "\n" ("Mide")) -> (w482:string)
                n183 = Get Date/Time In Seconds() -> (seconds since 1Jan1904=w496:timestamp)
                n184 = VISA Write(VISA resource name=w501, write buffer=w482, error in (no error)=w500) -> (VISA resource name out=w494:refnum<visa-resource-name>, error out=w493:errorcluster)  [unwired: 1 out]
                n185 = To Double Precision Float(number=w496) -> (double precision float=w495:dbl)
                n186 = while {
                  tunnel: w495 -> [w521]
                  shift-right: [w509] -> w491
                  shift-left: w494 -> [w520]
                  shift-right: [w508] -> w490
                  shift-left: w493 -> [w519]
                  tunnel: w492 -> [w517]
                  tunnel: [w516] -> _
                  shift-right: [w512] -> w488
                  shift-left: "" -> [w507]
                  stop <- w524 stop-if-true
                  n187 = Get Date/Time In Seconds() -> (seconds since 1Jan1904=w523:timestamp)
                  n188 = property class="Instr"(reference=w520, error in=w519) -> (reference out=w510:refnum<visa-resource-name>, error out=w511:errorcluster, "Serial Settings:Number of Bytes at Serial Port"=w514:u32)
                  n189 = To Double Precision Float(number=w523) -> (double precision float=w522:dbl)
                  n190 = Subtract(x=w522, y=w521) -> (x-y=w518:dbl)
                  n191 = Greater Than 0?(x=w514) -> (x > 0?=w513:bool)
                  n192 = case shown="True" w513 {
                    tunnel: w507 -> [w528 w533]
                    tunnel: [w528 w532] -> w512
                    tunnel: w511 -> [w526 w538]
                    tunnel: w510 -> [w525 w537]
                    tunnel: [w525 w536] -> w509
                    tunnel: [w526 w535] -> w508
                    tunnel: [FALSE w530] -> w506
                    frame False {
                    }
                    frame True {
                      n193 = local read "EOS"() -> (w529:string)
                      n194 = VISA Read(VISA resource name=w537, byte count=u32 1, error in (no error)=w538) -> (VISA resource name out=w536:refnum<visa-resource-name>, read buffer=w531:string, error out=w535:errorcluster)  [unwired: 1 out]
                      n195 = Equal?(x=w531, y=w529) -> (x = y?=w530:bool)
                      n196 = Concatenate Strings(w533, w531) -> (w532:string)
                    }
                  }
                  n197 = Greater Or Equal?(x=w518, y=w517) -> (x >= y?=w516:bool)
                  n198 = Or(x=w506, y=w516) -> (x .or. y?=w524:bool)
                  n199 = Wait (ms)(milliseconds to wait=u32 10) -> ()  [unwired: 1 out]
                }
                n200 = local write "read string"(w488) -> ()
              }
              frame "SET LIMITE PAR DE GIRO" {
                # "1.- Send command"
                # "3.- Wait for complet transmition"
                # "1.- Clear buffer"
                n201 = property class="Instr"(reference=w557, error in=w556) -> (reference out=w560:refnum<visa-resource-name>, error out=w561:errorcluster, "Serial Settings:Number of Bytes at Serial Port"=w562:u32)
                n202 = Number To Fractional String(number=w544, precision (6)=i16 3) -> (F-format string=w541:string)  [unwired: 2 in]
                n203 = VISA Read(VISA resource name=w560, byte count=w562, error in (no error)=w561) -> (VISA resource name out=w559:refnum<visa-resource-name>, error out=w558:errorcluster)  [unwired: 2 out]
                n204 = Concatenate Strings("OUT_SP_5 " ("Mide"), w541, "\n" ("Mide")) -> (w540:string)
                n205 = Get Date/Time In Seconds() -> (seconds since 1Jan1904=w554:timestamp)
                n206 = VISA Write(VISA resource name=w559, write buffer=w540, error in (no error)=w558) -> (VISA resource name out=w552:refnum<visa-resource-name>, error out=w551:errorcluster)  [unwired: 1 out]
                n207 = To Double Precision Float(number=w554) -> (double precision float=w553:dbl)
                n208 = while {
                  tunnel: w553 -> [w579]
                  shift-right: [w567] -> w549
                  shift-left: w552 -> [w578]
                  shift-right: [w566] -> w548
                  shift-left: w551 -> [w577]
                  tunnel: w550 -> [w575]
                  tunnel: [w574] -> _
                  shift-right: [w570] -> w546
                  shift-left: "" -> [w565]
                  stop <- w582 stop-if-true
                  n209 = Get Date/Time In Seconds() -> (seconds since 1Jan1904=w581:timestamp)
                  n210 = property class="Instr"(reference=w578, error in=w577) -> (reference out=w568:refnum<visa-resource-name>, error out=w569:errorcluster, "Serial Settings:Number of Bytes at Serial Port"=w572:u32)
                  n211 = To Double Precision Float(number=w581) -> (double precision float=w580:dbl)
                  n212 = Subtract(x=w580, y=w579) -> (x-y=w576:dbl)
                  n213 = Greater Than 0?(x=w572) -> (x > 0?=w571:bool)
                  n214 = case shown="True" w571 {
                    tunnel: w565 -> [w586 w591]
                    tunnel: [w586 w590] -> w570
                    tunnel: w569 -> [w584 w596]
                    tunnel: w568 -> [w583 w595]
                    tunnel: [w583 w594] -> w567
                    tunnel: [w584 w593] -> w566
                    tunnel: [FALSE w588] -> w564
                    frame False {
                    }
                    frame True {
                      n215 = local read "EOS"() -> (w587:string)
                      n216 = VISA Read(VISA resource name=w595, byte count=u32 1, error in (no error)=w596) -> (VISA resource name out=w594:refnum<visa-resource-name>, read buffer=w589:string, error out=w593:errorcluster)  [unwired: 1 out]
                      n217 = Equal?(x=w589, y=w587) -> (x = y?=w588:bool)
                      n218 = Concatenate Strings(w591, w589) -> (w590:string)
                    }
                  }
                  n219 = Greater Or Equal?(x=w576, y=w575) -> (x >= y?=w574:bool)
                  n220 = Or(x=w564, y=w574) -> (x .or. y?=w582:bool)
                  n221 = Wait (ms)(milliseconds to wait=u32 10) -> ()  [unwired: 1 out]
                }
                n222 = local write "read string"(w546) -> ()
              }
              frame "SET LIMITE VELOCIDAD" {
                # "1.- Send command"
                # "3.- Wait for complet transmition"
                # "1.- Clear buffer"
                n223 = property class="Instr"(reference=w615, error in=w614) -> (reference out=w618:refnum<visa-resource-name>, error out=w619:errorcluster, "Serial Settings:Number of Bytes at Serial Port"=w620:u32)
                n224 = Number To Fractional String(number=w602, precision (6)=i16 3) -> (F-format string=w599:string)  [unwired: 2 in]
                n225 = VISA Read(VISA resource name=w618, byte count=w620, error in (no error)=w619) -> (VISA resource name out=w617:refnum<visa-resource-name>, error out=w616:errorcluster)  [unwired: 2 out]
                n226 = Concatenate Strings("OUT_SP_6 " ("Mide"), w599, "\n" ("Mide")) -> (w598:string)
                n227 = Get Date/Time In Seconds() -> (seconds since 1Jan1904=w612:timestamp)
                n228 = VISA Write(VISA resource name=w617, write buffer=w598, error in (no error)=w616) -> (VISA resource name out=w610:refnum<visa-resource-name>, error out=w609:errorcluster)  [unwired: 1 out]
                n229 = To Double Precision Float(number=w612) -> (double precision float=w611:dbl)
                n230 = while {
                  tunnel: w611 -> [w637]
                  shift-right: [w625] -> w607
                  shift-left: w610 -> [w636]
                  shift-right: [w624] -> w606
                  shift-left: w609 -> [w635]
                  tunnel: w608 -> [w633]
                  tunnel: [w632] -> _
                  shift-right: [w628] -> w604
                  shift-left: "" -> [w623]
                  stop <- w640 stop-if-true
                  n231 = Get Date/Time In Seconds() -> (seconds since 1Jan1904=w639:timestamp)
                  n232 = property class="Instr"(reference=w636, error in=w635) -> (reference out=w626:refnum<visa-resource-name>, error out=w627:errorcluster, "Serial Settings:Number of Bytes at Serial Port"=w630:u32)
                  n233 = To Double Precision Float(number=w639) -> (double precision float=w638:dbl)
                  n234 = Subtract(x=w638, y=w637) -> (x-y=w634:dbl)
                  n235 = Greater Than 0?(x=w630) -> (x > 0?=w629:bool)
                  n236 = case shown="True" w629 {
                    tunnel: w623 -> [w644 w649]
                    tunnel: [w644 w648] -> w628
                    tunnel: w627 -> [w642 w654]
                    tunnel: w626 -> [w641 w653]
                    tunnel: [w641 w652] -> w625
                    tunnel: [w642 w651] -> w624
                    tunnel: [FALSE w646] -> w622
                    frame False {
                    }
                    frame True {
                      n237 = local read "EOS"() -> (w645:string)
                      n238 = VISA Read(VISA resource name=w653, byte count=u32 1, error in (no error)=w654) -> (VISA resource name out=w652:refnum<visa-resource-name>, read buffer=w647:string, error out=w651:errorcluster)  [unwired: 1 out]
                      n239 = Equal?(x=w647, y=w645) -> (x = y?=w646:bool)
                      n240 = Concatenate Strings(w649, w647) -> (w648:string)
                    }
                  }
                  n241 = Greater Or Equal?(x=w634, y=w633) -> (x >= y?=w632:bool)
                  n242 = Or(x=w622, y=w632) -> (x .or. y?=w640:bool)
                  n243 = Wait (ms)(milliseconds to wait=u32 10) -> ()  [unwired: 1 out]
                }
                n244 = local write "read string"(w604) -> ()
              }
              frame "SET VELOCIDAD SEGURIDAD" {
                # "1.- Send command"
                # "3.- Wait for complet transmition"
                # "1.- Clear buffer"
                n245 = property class="Instr"(reference=w673, error in=w672) -> (reference out=w676:refnum<visa-resource-name>, error out=w677:errorcluster, "Serial Settings:Number of Bytes at Serial Port"=w678:u32)
                n246 = Number To Fractional String(number=w660, precision (6)=i16 3) -> (F-format string=w657:string)  [unwired: 2 in]
                n247 = VISA Read(VISA resource name=w676, byte count=w678, error in (no error)=w677) -> (VISA resource name out=w675:refnum<visa-resource-name>, error out=w674:errorcluster)  [unwired: 2 out]
                n248 = Concatenate Strings("OUT_SP_8 " ("Mide"), w657, "\n" ("Mide")) -> (w656:string)
                n249 = Get Date/Time In Seconds() -> (seconds since 1Jan1904=w670:timestamp)
                n250 = VISA Write(VISA resource name=w675, write buffer=w656, error in (no error)=w674) -> (VISA resource name out=w668:refnum<visa-resource-name>, error out=w667:errorcluster)  [unwired: 1 out]
                n251 = To Double Precision Float(number=w670) -> (double precision float=w669:dbl)
                n252 = while {
                  tunnel: w669 -> [w695]
                  shift-right: [w683] -> w665
                  shift-left: w668 -> [w694]
                  shift-right: [w682] -> w664
                  shift-left: w667 -> [w693]
                  tunnel: w666 -> [w691]
                  tunnel: [w690] -> _
                  shift-right: [w686] -> w662
                  shift-left: "" -> [w681]
                  stop <- w698 stop-if-true
                  n253 = Get Date/Time In Seconds() -> (seconds since 1Jan1904=w697:timestamp)
                  n254 = property class="Instr"(reference=w694, error in=w693) -> (reference out=w684:refnum<visa-resource-name>, error out=w685:errorcluster, "Serial Settings:Number of Bytes at Serial Port"=w688:u32)
                  n255 = To Double Precision Float(number=w697) -> (double precision float=w696:dbl)
                  n256 = Subtract(x=w696, y=w695) -> (x-y=w692:dbl)
                  n257 = Greater Than 0?(x=w688) -> (x > 0?=w687:bool)
                  n258 = case shown="True" w687 {
                    tunnel: w681 -> [w702 w707]
                    tunnel: [w702 w706] -> w686
                    tunnel: w685 -> [w700 w712]
                    tunnel: w684 -> [w699 w711]
                    tunnel: [w699 w710] -> w683
                    tunnel: [w700 w709] -> w682
                    tunnel: [FALSE w704] -> w680
                    frame False {
                    }
                    frame True {
                      n259 = local read "EOS"() -> (w703:string)
                      n260 = VISA Read(VISA resource name=w711, byte count=u32 1, error in (no error)=w712) -> (VISA resource name out=w710:refnum<visa-resource-name>, read buffer=w705:string, error out=w709:errorcluster)  [unwired: 1 out]
                      n261 = Equal?(x=w705, y=w703) -> (x = y?=w704:bool)
                      n262 = Concatenate Strings(w707, w705) -> (w706:string)
                    }
                  }
                  n263 = Greater Or Equal?(x=w692, y=w691) -> (x >= y?=w690:bool)
                  n264 = Or(x=w680, y=w690) -> (x .or. y?=w698:bool)
                  n265 = Wait (ms)(milliseconds to wait=u32 10) -> ()  [unwired: 1 out]
                }
                n266 = local write "read string"(w662) -> ()
              }
              frame "ARRANCAR MOTOR" {
                w714 = "START_4\n" ("Mide")
                # "1.- Send command"
                # "3.- Wait for complet transmition"
                # "1.- Clear buffer"
                n267 = property class="Instr"(reference=w730, error in=w729) -> (reference out=w733:refnum<visa-resource-name>, error out=w734:errorcluster, "Serial Settings:Number of Bytes at Serial Port"=w735:u32)
                n268 = Number To Fractional String(number=w717, precision (6)=i16 3) -> (F-format string=w715:string)  [unwired: 2 in]
                n269 = VISA Read(VISA resource name=w733, byte count=w735, error in (no error)=w734) -> (VISA resource name out=w732:refnum<visa-resource-name>, error out=w731:errorcluster)  [unwired: 2 out]
                n270 = Concatenate Strings(w714, w715, "\n" ("Mide")) -> ()  [unwired: 1 out]
                n271 = Get Date/Time In Seconds() -> (seconds since 1Jan1904=w727:timestamp)
                n272 = VISA Write(VISA resource name=w732, write buffer=w714, error in (no error)=w731) -> (VISA resource name out=w725:refnum<visa-resource-name>, error out=w724:errorcluster)  [unwired: 1 out]
                n273 = To Double Precision Float(number=w727) -> (double precision float=w726:dbl)
                n274 = while {
                  tunnel: w726 -> [w752]
                  shift-right: [w740] -> w722
                  shift-left: w725 -> [w751]
                  shift-right: [w739] -> w721
                  shift-left: w724 -> [w750]
                  tunnel: w723 -> [w748]
                  tunnel: [w747] -> _
                  shift-right: [w743] -> w719
                  shift-left: "" -> [w738]
                  stop <- w755 stop-if-true
                  n275 = Get Date/Time In Seconds() -> (seconds since 1Jan1904=w754:timestamp)
                  n276 = property class="Instr"(reference=w751, error in=w750) -> (reference out=w741:refnum<visa-resource-name>, error out=w742:errorcluster, "Serial Settings:Number of Bytes at Serial Port"=w745:u32)
                  n277 = To Double Precision Float(number=w754) -> (double precision float=w753:dbl)
                  n278 = Subtract(x=w753, y=w752) -> (x-y=w749:dbl)
                  n279 = Greater Than 0?(x=w745) -> (x > 0?=w744:bool)
                  n280 = case shown="True" w744 {
                    tunnel: w738 -> [w759 w764]
                    tunnel: [w759 w763] -> w743
                    tunnel: w742 -> [w757 w769]
                    tunnel: w741 -> [w756 w768]
                    tunnel: [w756 w767] -> w740
                    tunnel: [w757 w766] -> w739
                    tunnel: [FALSE w761] -> w737
                    frame False {
                    }
                    frame True {
                      n281 = local read "EOS"() -> (w760:string)
                      n282 = VISA Read(VISA resource name=w768, byte count=u32 1, error in (no error)=w769) -> (VISA resource name out=w767:refnum<visa-resource-name>, read buffer=w762:string, error out=w766:errorcluster)  [unwired: 1 out]
                      n283 = Equal?(x=w762, y=w760) -> (x = y?=w761:bool)
                      n284 = Concatenate Strings(w764, w762) -> (w763:string)
                    }
                  }
                  n285 = Greater Or Equal?(x=w749, y=w748) -> (x >= y?=w747:bool)
                  n286 = Or(x=w737, y=w747) -> (x .or. y?=w755:bool)
                  n287 = Wait (ms)(milliseconds to wait=u32 10) -> ()  [unwired: 1 out]
                }
                n288 = local write "read string"(w719) -> ()
              }
              frame "DETENER MOTOR" {
                w771 = "STOP_4\n" ("Mide")
                # "1.- Send command"
                # "3.- Wait for complet transmition"
                # "1.- Clear buffer"
                n289 = property class="Instr"(reference=w787, error in=w786) -> (reference out=w790:refnum<visa-resource-name>, error out=w791:errorcluster, "Serial Settings:Number of Bytes at Serial Port"=w792:u32)
                n290 = Number To Fractional String(number=w774, precision (6)=i16 3) -> (F-format string=w772:string)  [unwired: 2 in]
                n291 = VISA Read(VISA resource name=w790, byte count=w792, error in (no error)=w791) -> (VISA resource name out=w789:refnum<visa-resource-name>, error out=w788:errorcluster)  [unwired: 2 out]
                n292 = Concatenate Strings(w771, w772, "\n" ("Mide")) -> ()  [unwired: 1 out]
                n293 = Get Date/Time In Seconds() -> (seconds since 1Jan1904=w784:timestamp)
                n294 = VISA Write(VISA resource name=w789, write buffer=w771, error in (no error)=w788) -> (VISA resource name out=w782:refnum<visa-resource-name>, error out=w781:errorcluster)  [unwired: 1 out]
                n295 = To Double Precision Float(number=w784) -> (double precision float=w783:dbl)
                n296 = while {
                  tunnel: w783 -> [w809]
                  shift-right: [w797] -> w779
                  shift-left: w782 -> [w808]
                  shift-right: [w796] -> w778
                  shift-left: w781 -> [w807]
                  tunnel: w780 -> [w805]
                  tunnel: [w804] -> _
                  shift-right: [w800] -> w776
                  shift-left: "" -> [w795]
                  stop <- w812 stop-if-true
                  n297 = Get Date/Time In Seconds() -> (seconds since 1Jan1904=w811:timestamp)
                  n298 = property class="Instr"(reference=w808, error in=w807) -> (reference out=w798:refnum<visa-resource-name>, error out=w799:errorcluster, "Serial Settings:Number of Bytes at Serial Port"=w802:u32)
                  n299 = To Double Precision Float(number=w811) -> (double precision float=w810:dbl)
                  n300 = Subtract(x=w810, y=w809) -> (x-y=w806:dbl)
                  n301 = Greater Than 0?(x=w802) -> (x > 0?=w801:bool)
                  n302 = case shown="True" w801 {
                    tunnel: w795 -> [w816 w821]
                    tunnel: [w816 w820] -> w800
                    tunnel: w799 -> [w814 w826]
                    tunnel: w798 -> [w813 w825]
                    tunnel: [w813 w824] -> w797
                    tunnel: [w814 w823] -> w796
                    tunnel: [FALSE w818] -> w794
                    frame False {
                    }
                    frame True {
                      n303 = local read "EOS"() -> (w817:string)
                      n304 = VISA Read(VISA resource name=w825, byte count=u32 1, error in (no error)=w826) -> (VISA resource name out=w824:refnum<visa-resource-name>, read buffer=w819:string, error out=w823:errorcluster)  [unwired: 1 out]
                      n305 = Equal?(x=w819, y=w817) -> (x = y?=w818:bool)
                      n306 = Concatenate Strings(w821, w819) -> (w820:string)
                    }
                  }
                  n307 = Greater Or Equal?(x=w806, y=w805) -> (x >= y?=w804:bool)
                  n308 = Or(x=w794, y=w804) -> (x .or. y?=w812:bool)
                  n309 = Wait (ms)(milliseconds to wait=u32 10) -> ()  [unwired: 1 out]
                }
                n310 = local write "read string"(w776) -> ()
              }
              frame "RESET" {
                w828 = "RESET\n" ("Mide")
                # "1.- Send command"
                # "3.- Wait for complet transmition"
                # "1.- Clear buffer"
                n311 = property class="Instr"(reference=w844, error in=w843) -> (reference out=w847:refnum<visa-resource-name>, error out=w848:errorcluster, "Serial Settings:Number of Bytes at Serial Port"=w849:u32)
                n312 = Number To Fractional String(number=w831, precision (6)=i16 3) -> (F-format string=w829:string)  [unwired: 2 in]
                n313 = VISA Read(VISA resource name=w847, byte count=w849, error in (no error)=w848) -> (VISA resource name out=w846:refnum<visa-resource-name>, error out=w845:errorcluster)  [unwired: 2 out]
                n314 = Concatenate Strings(w828, w829, "\n" ("Mide")) -> ()  [unwired: 1 out]
                n315 = Get Date/Time In Seconds() -> (seconds since 1Jan1904=w841:timestamp)
                n316 = VISA Write(VISA resource name=w846, write buffer=w828, error in (no error)=w845) -> (VISA resource name out=w839:refnum<visa-resource-name>, error out=w838:errorcluster)  [unwired: 1 out]
                n317 = To Double Precision Float(number=w841) -> (double precision float=w840:dbl)
                n318 = while {
                  tunnel: w840 -> [w866]
                  shift-right: [w854] -> w836
                  shift-left: w839 -> [w865]
                  shift-right: [w853] -> w835
                  shift-left: w838 -> [w864]
                  tunnel: w837 -> [w862]
                  tunnel: [w861] -> _
                  shift-right: [w857] -> w833
                  shift-left: "" -> [w852]
                  stop <- w869 stop-if-true
                  n319 = Get Date/Time In Seconds() -> (seconds since 1Jan1904=w868:timestamp)
                  n320 = property class="Instr"(reference=w865, error in=w864) -> (reference out=w855:refnum<visa-resource-name>, error out=w856:errorcluster, "Serial Settings:Number of Bytes at Serial Port"=w859:u32)
                  n321 = To Double Precision Float(number=w868) -> (double precision float=w867:dbl)
                  n322 = Subtract(x=w867, y=w866) -> (x-y=w863:dbl)
                  n323 = Greater Than 0?(x=w859) -> (x > 0?=w858:bool)
                  n324 = case shown="True" w858 {
                    tunnel: w852 -> [w873 w878]
                    tunnel: [w873 w877] -> w857
                    tunnel: w856 -> [w871 w883]
                    tunnel: w855 -> [w870 w882]
                    tunnel: [w870 w881] -> w854
                    tunnel: [w871 w880] -> w853
                    tunnel: [FALSE w875] -> w851
                    frame False {
                    }
                    frame True {
                      n325 = local read "EOS"() -> (w874:string)
                      n326 = VISA Read(VISA resource name=w882, byte count=u32 1, error in (no error)=w883) -> (VISA resource name out=w881:refnum<visa-resource-name>, read buffer=w876:string, error out=w880:errorcluster)  [unwired: 1 out]
                      n327 = Equal?(x=w876, y=w874) -> (x = y?=w875:bool)
                      n328 = Concatenate Strings(w878, w876) -> (w877:string)
                    }
                  }
                  n329 = Greater Or Equal?(x=w863, y=w862) -> (x >= y?=w861:bool)
                  n330 = Or(x=w851, y=w861) -> (x .or. y?=w869:bool)
                  n331 = Wait (ms)(milliseconds to wait=u32 10) -> ()  [unwired: 1 out]
                }
                n332 = local write "read string"(w833) -> ()
              }
              frame "SET SENTIDO DE GIRO" {
                # "1.- Send command"
                # "3.- Wait for complet transmition"
                # "1.- Clear buffer"
                n333 = property class="Instr"(reference=w902, error in=w901) -> (reference out=w905:refnum<visa-resource-name>, error out=w906:errorcluster, "Serial Settings:Number of Bytes at Serial Port"=w907:u32)
                n334 = To Byte Integer(number=w888) -> (8bit integer=w887:i8)
                n335 = Number To Decimal String(number=w887) -> (decimal integer string=w889:string)  [unwired: 1 in]
                n336 = VISA Read(VISA resource name=w905, byte count=w907, error in (no error)=w906) -> (VISA resource name out=w904:refnum<visa-resource-name>, error out=w903:errorcluster)  [unwired: 2 out]
                n337 = Concatenate Strings("OUT_MODE_" ("Mide"), w889, "\n" ("Mide")) -> (w885:string)
                n338 = Get Date/Time In Seconds() -> (seconds since 1Jan1904=w899:timestamp)
                n339 = VISA Write(VISA resource name=w904, write buffer=w885, error in (no error)=w903) -> (VISA resource name out=w897:refnum<visa-resource-name>, error out=w896:errorcluster)  [unwired: 1 out]
                n340 = To Double Precision Float(number=w899) -> (double precision float=w898:dbl)
                n341 = while {
                  tunnel: w898 -> [w924]
                  shift-right: [w912] -> w894
                  shift-left: w897 -> [w923]
                  shift-right: [w911] -> w893
                  shift-left: w896 -> [w922]
                  tunnel: w895 -> [w920]
                  tunnel: [w919] -> _
                  shift-right: [w915] -> w891
                  shift-left: "" -> [w910]
                  stop <- w927 stop-if-true
                  n342 = Get Date/Time In Seconds() -> (seconds since 1Jan1904=w926:timestamp)
                  n343 = property class="Instr"(reference=w923, error in=w922) -> (reference out=w913:refnum<visa-resource-name>, error out=w914:errorcluster, "Serial Settings:Number of Bytes at Serial Port"=w917:u32)
                  n344 = To Double Precision Float(number=w926) -> (double precision float=w925:dbl)
                  n345 = Subtract(x=w925, y=w924) -> (x-y=w921:dbl)
                  n346 = Greater Than 0?(x=w917) -> (x > 0?=w916:bool)
                  n347 = case shown="True" w916 {
                    tunnel: w910 -> [w931 w936]
                    tunnel: [w931 w935] -> w915
                    tunnel: w914 -> [w929 w941]
                    tunnel: w913 -> [w928 w940]
                    tunnel: [w928 w939] -> w912
                    tunnel: [w929 w938] -> w911
                    tunnel: [FALSE w933] -> w909
                    frame False {
                    }
                    frame True {
                      n348 = local read "EOS"() -> (w932:string)
                      n349 = VISA Read(VISA resource name=w940, byte count=u32 1, error in (no error)=w941) -> (VISA resource name out=w939:refnum<visa-resource-name>, read buffer=w934:string, error out=w938:errorcluster)  [unwired: 1 out]
                      n350 = Equal?(x=w934, y=w932) -> (x = y?=w933:bool)
                      n351 = Concatenate Strings(w936, w934) -> (w935:string)
                    }
                  }
                  n352 = Greater Or Equal?(x=w921, y=w920) -> (x >= y?=w919:bool)
                  n353 = Or(x=w909, y=w919) -> (x .or. y?=w927:bool)
                  n354 = Wait (ms)(milliseconds to wait=u32 10) -> ()  [unwired: 1 out]
                }
                n355 = local write "read string"(w891) -> ()
              }
              frame "READ SENTIDO DE GIRO" {
                (unwired) "IN_MODE %f" ("format string")
                w945 = "IN_MODE\n" ("Mide")
                # "1.- Send command"
                # "3.- Wait for complet transmition"
                # "1.- Clear buffer"
                n356 = property class="Instr"(reference=w960, error in=w959) -> (reference out=w963:refnum<visa-resource-name>, error out=w964:errorcluster, "Serial Settings:Number of Bytes at Serial Port"=w965:u32)
                n357 = To Byte Integer(number=w947) -> (8bit integer=w946:i8)
                n358 = Number To Decimal String(number=w946) -> (decimal integer string=w948:string)  [unwired: 1 in]
                n359 = VISA Read(VISA resource name=w963, byte count=w965, error in (no error)=w964) -> (VISA resource name out=w962:refnum<visa-resource-name>, error out=w961:errorcluster)  [unwired: 2 out]
                n360 = Concatenate Strings(w945, w948, "\n" ("Mide")) -> ()  [unwired: 1 out]
                n361 = Get Date/Time In Seconds() -> (seconds since 1Jan1904=w957:timestamp)
                n362 = VISA Write(VISA resource name=w962, write buffer=w945, error in (no error)=w961) -> (VISA resource name out=w955:refnum<visa-resource-name>, error out=w954:errorcluster)  [unwired: 1 out]
                n363 = To Double Precision Float(number=w957) -> (double precision float=w956:dbl)
                n364 = while {
                  tunnel: w956 -> [w982]
                  shift-right: [w970] -> w952
                  shift-left: w955 -> [w981]
                  shift-right: [w969] -> w951
                  shift-left: w954 -> [w980]
                  tunnel: w953 -> [w978]
                  tunnel: [w977] -> _
                  shift-right: [w973] -> w943
                  shift-left: "" -> [w968]
                  stop <- w985 stop-if-true
                  n365 = Get Date/Time In Seconds() -> (seconds since 1Jan1904=w984:timestamp)
                  n366 = property class="Instr"(reference=w981, error in=w980) -> (reference out=w971:refnum<visa-resource-name>, error out=w972:errorcluster, "Serial Settings:Number of Bytes at Serial Port"=w975:u32)
                  n367 = To Double Precision Float(number=w984) -> (double precision float=w983:dbl)
                  n368 = Subtract(x=w983, y=w982) -> (x-y=w979:dbl)
                  n369 = Greater Than 0?(x=w975) -> (x > 0?=w974:bool)
                  n370 = case shown="True" w974 {
                    tunnel: w968 -> [w989 w994]
                    tunnel: [w989 w993] -> w973
                    tunnel: w972 -> [w987 w999]
                    tunnel: w971 -> [w986 w998]
                    tunnel: [w986 w997] -> w970
                    tunnel: [w987 w996] -> w969
                    tunnel: [FALSE w991] -> w967
                    frame False {
                    }
                    frame True {
                      n371 = local read "EOS"() -> (w990:string)
                      n372 = VISA Read(VISA resource name=w998, byte count=u32 1, error in (no error)=w999) -> (VISA resource name out=w997:refnum<visa-resource-name>, read buffer=w992:string, error out=w996:errorcluster)  [unwired: 1 out]
                      n373 = Equal?(x=w992, y=w990) -> (x = y?=w991:bool)
                      n374 = Concatenate Strings(w994, w992) -> (w993:string)
                    }
                  }
                  n375 = Greater Or Equal?(x=w979, y=w978) -> (x >= y?=w977:bool)
                  n376 = Or(x=w967, y=w977) -> (x .or. y?=w985:bool)
                  n377 = Wait (ms)(milliseconds to wait=u32 10) -> ()  [unwired: 1 out]
                }
                n378 = Scan Value(string=w943, format string="%f") -> (value=w942:dbl)  [unwired: 1 in, 1 out]
                n379 = local write "read string"(w943) -> ()
              }
              frame "FINALIZAR" {
                n380 = VISA Close(VISA resource name=w1002, error in (no error)=w1004) -> (error out=w1003:errorcluster)
              }
            }
            "Read_parametro" <- w16
          }
        }
        frame Error {
        }
      }
    }
  }
  "error out" <- w2
